vi "Basic Set Valve Position.vi"() -> ()   [LabVIEW 2016]
doc: "Purpose: This example shows how to change the position of a valve \n\nHardware setup: at least one Fluigent valve controller (M-Switch, L-Switch, 2-Switch or P-Switch)"
uses:
  fgt_SDK.lvlib
panel:
  out "Current position":i32
  in  "valveIndex":u32
  in  "Target position":i32(slide) min=0 max=9 step=1 scale=0.0..9.0
  in  "Stop button":bool
  out "error out":errorcluster
  # "Select a valve index and set its position"
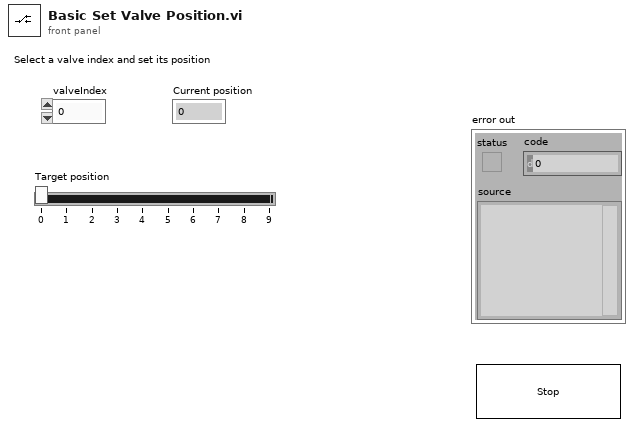
[diagram p1: front panel]
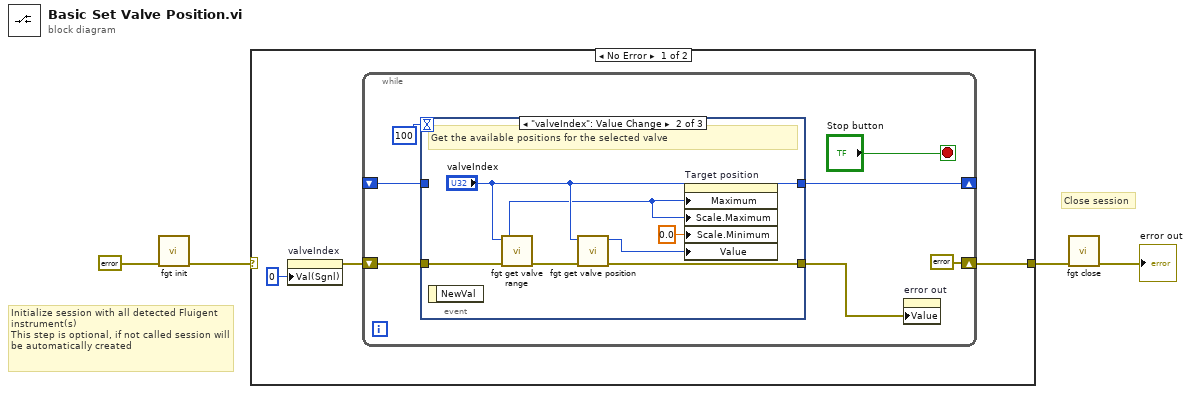
[diagram p0: block diagram]
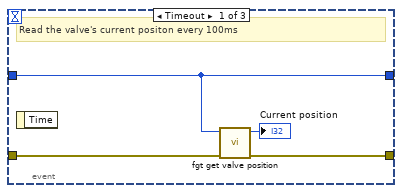
[diagram p2: hidden frame]
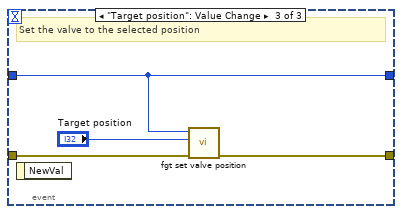
[diagram p3: hidden frame]
diagram:
  # "Close session"
  # "Initialize session with all detected Fluigent instrument(s)\nThis step is optional, if not called session will be automatically created"
  n1 = call "fgt init.vi"("error in (no error)"=errorcluster {"status"=FALSE, "code"=0, "source"=""}) -> ("error out"=w4:errorcluster)  [unwired: 10 in]
  n2 = case shown="No Error" w4 {
    selector: w4 -> [_ w29]
    tunnel: [w7 w29] -> w2
    frame No Error {
      n3 = property on="valveIndex" class="DigNum (strict)"("Val(Sgnl)"=u32 0 ("Value (Signaling)")) -> (error out=w6:errorcluster)  [unwired: 2 in, 1 out]
      n4 = while {
        shift-right: [errorcluster {"status"=FALSE, "code"=0, "source"=""} ("error out")] -> w7
        shift-left: w6 -> [w12]
        shift-right: [w10] -> _
        shift-left: _ -> [w9]
        stop <- "Stop button" stop-if-true
        n5 = event shown="[1] \"valveIndex\": Value Change" {
          selector: _ -> [_ _ _]
          dyn-events: _ -> [_ _ _]
          timeout: 100 -> [_ _ _]
          tunnel: w12 -> [w18 w24 w28]
          tunnel: [w16 w23 w27] -> w8
          tunnel: [w15 "valveIndex" w26] -> w10
          tunnel: w9 -> [w15 _ w26]
          event Timeout {
            # "Read the valve's current positon every 100ms"
            n6 = event-data() -> ()  [unwired: 1 in, 1 out]
            n7 = call "fgt get valve position.vi"("error in (no error)"=w18, "valveIndex"=w15) -> ("error out"=w16:errorcluster, "position"=→"Current position":i32)  [unwired: 8 in]
          }
          event "valveIndex": Value Change {
            # "Get the available positions for the selected valve"
            n8 = event-data() -> ()  [unwired: 1 in, 1 out]
            n9 = call "fgt get valve range.vi"("error in (no error)"=w24, "valveIndex"="valveIndex") -> ("max position"=w20:i32)  [unwired: 8 in, 1 out]
            n10 = call "fgt get valve position.vi"("error in (no error)"=w24, "valveIndex"="valveIndex") -> ("error out"=w23:errorcluster, "position"=w21:i32)  [unwired: 8 in]
            n11 = property on="Target position" class="Slide (strict)"("Maximum"=w20, "Scale.Maximum"=w20, "Scale.Minimum"=0.0 ("Scale.Range:Minimum"), "Value"=w21) -> ()  [unwired: 2 in, 2 out]
          }
          event "Target position": Value Change {
            # "Set the valve to the selected position"
            n12 = event-data() -> ()  [unwired: 1 in, 1 out]
            n13 = call "fgt set valve position.vi"("error in (no error)"=w28, "position"="Target position", "valveIndex"=w26) -> ("error out"=w27:errorcluster)  [unwired: 8 in]
          }
        }
        n14 = property on="error out" class="Clust (strict)"("Value"=w8) -> ()  [unwired: 2 in, 2 out]
      }
    }
    frame Error {
    }
  }
  n15 = call "fgt close.vi"("error in (no error)"=w2) -> ("error out"=→"error out":errorcluster)  [unwired: 10 in]
